vi "breakIn_toplvl_zapOption-v01.vi"(0 "Pressure box control in":T3={"Pressure box COM"="COM7", "pressure box type"=enum."ProportionAir", "High pos pressure (mBar)"=0.0, "Low pos pressure (mBar)"=0.0, "Vacuum pressure (mBar)"=0.0, "calibration"=enum."mightenRig"}, 1 "Multiclamp Handle In":u32=722860, 3 "which manipulator":T2(ring), 5 "break in duration (ms)":i32(knob)=100 min=50 max=2000 step=50 scale=0.0..2000.0, 7 "mclamp cluster":T1, 9 "give a zap?":bool, 11 "error in (no error)":errorcluster) -> (4 "Pressure box control out":T3, 15 "error out":errorcluster)   [LabVIEW 2015]
uses:
  controls/proportionAir_cmds.ctl
  controls/arduino_pressure_setting.ctl
  multiBot/patcherBot/AxMultiClampMsg.dll
  controls/pressure_box_type.ctl
  controls/pressure_box_control.ctl
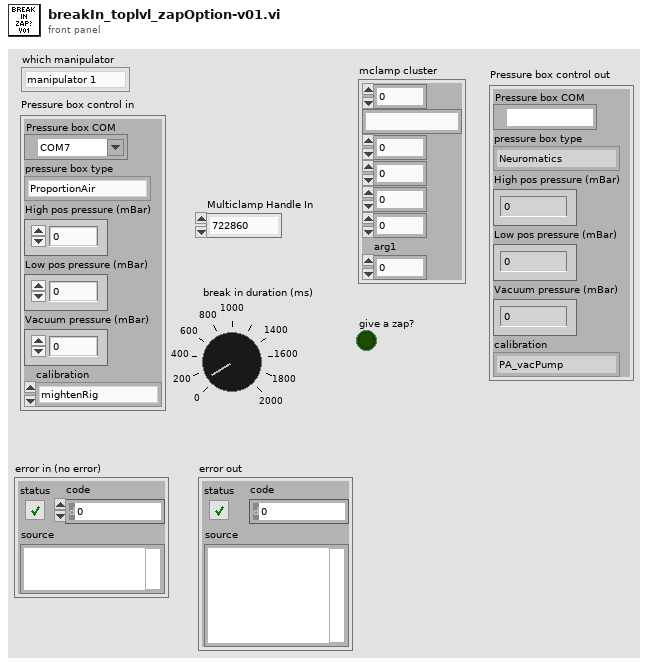
[diagram p1: front panel]
types:
  T1 = cluster{u32, string, i32, u32, u32, u32, "arg1":i32}
  T2 = enum16{"manipulator 1", "manipulator 2", "manipulator 3", "manipulator 4"}
  T3 = typedef "pressure_box_control.ctl" = cluster{"Pressure box COM":refnum<visa-resource-name>, "pressure box type":T4, "High pos pressure (mBar)":dbl, "Low pos pressure (mBar)":dbl, "Vacuum pressure (mBar)":dbl, "calibration":enum16{"PA_vacPump", "PA_venturi", "Neuromatics", "ilyaRig", "mightenRig"}}
  T4 = typedef "pressure_box_type.ctl" = enum16{"Neuromatics", "ProportionAir", "Demo box", "N-ProportionAir"}
  T5 = typedef "proportionAir_cmds.ctl" = enum16{"Set P", "Switch to Atm", "Switch to Regulator", "Pulse", "WC"}
  T6 = typedef "arduino_pressure_setting.ctl" = enum16{"High Positive Pressure", "Low Positive Pressure", "Atmospheric Pressure", "Low Vacuum", "High Vacuum", "Break In", "Puff"}
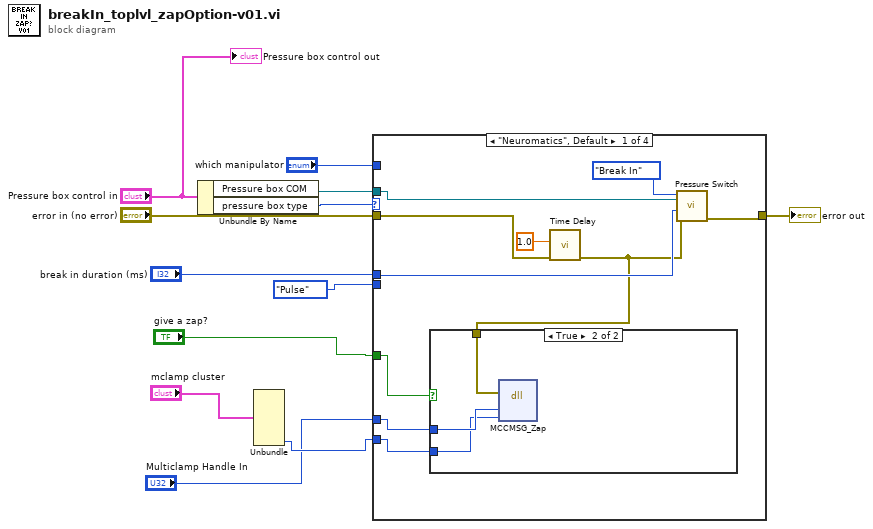
[diagram p0: block diagram]
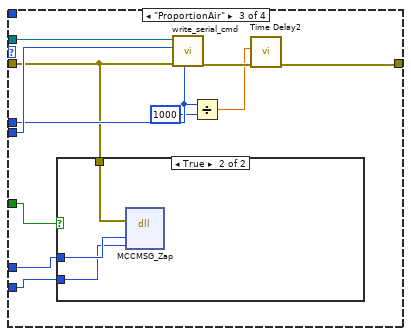
[diagram p4: hidden frame]
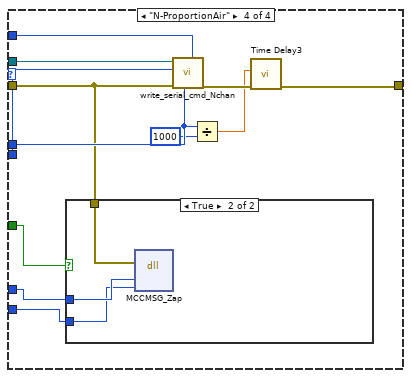
[diagram p6: hidden frame]
diagram:
  n1 = Unbundle By Name("Pressure box control in") -> ("Pressure box COM"=w10:refnum<visa-resource-name>, "pressure box type"=w11:T4)
  n2 = Unbundle("mclamp cluster") -> ("arg1"=w2:i32)  [unwired: 6 out]
  n3 = case shown="\"Neuromatics\", Default" w11 {
    tunnel: "error in (no error)" -> [w17 w26 w27 w41]
    tunnel: [w22 w26 w34 w49] -> w9
    tunnel: w10 -> [w18 _ w37 w52]
    tunnel: proportionAir_cmds."Pulse" ("pressure command") -> [_ _ w36 w51]
    tunnel: "break in duration (ms)" -> [w21 _ w33 w48]
    tunnel: "which manipulator" -> [_ _ _ w45]
    tunnel: "give a zap?" -> [w16 _ w28 w44]
    tunnel: w2 -> [w14 _ w29 w42]
    tunnel: "Multiclamp Handle In" -> [w15 _ w30 w43]
    frame "Neuromatics", Default {
      n4 = call "Time Delay"("error in (no error)"=w17, "Delay Time (s)"=1.0) -> ("error out"=w13:errorcluster)  [unwired: 9 in]
      n5 = case shown="True" w16 {
        tunnel: w15 -> [_ w25]
        tunnel: w14 -> [_ w24]
        tunnel: w13 -> [_ w23]
        frame False {
        }
        frame True {
          n6 = dll-call lib="C:/multiBot/patcherBot/AxMultiClampMsg.dll" fn="MCCMSG_Zap"(error in=w23, "handle"=w25, "error"=w24) -> ()  [unwired: 5 in, 2 out]
        }
      }
      n7 = call "Pressure Switch.vi"("error in"=w13, "Break In Time"=w21, "Pressure Box COM"=w18, "arduino pressure setting"=arduino_pressure_setting."Break In") -> ("error out"=w22:errorcluster)  [unwired: 6 in, 1 out]
    }
    frame "Demo box" {
    }
    frame "ProportionAir" {
      n8 = case shown="True" w28 {
        tunnel: w30 -> [_ w40]
        tunnel: w29 -> [_ w39]
        tunnel: w27 -> [_ w38]
        frame False {
        }
        frame True {
          n9 = dll-call lib="C:/multiBot/patcherBot/AxMultiClampMsg.dll" fn="MCCMSG_Zap"(error in=w38, "handle"=w40, "error"=w39) -> ()  [unwired: 5 in, 2 out]
        }
      }
      n10 = call "write_serial_cmd.vi"("pulse duration (ms)"=w33, "error in"=w27, "pressure command"=w36, "Pressure Box COM"=w37) -> ("error out"=w35:errorcluster)  [unwired: 6 in, 1 out]
      n11 = Divide(x=w33, y=1000) -> (x/y=w31:dbl)
      n12 = call "Time Delay2"("error in (no error)"=w35, "Delay Time (s)"=w31) -> ("error out"=w34:errorcluster)  [unwired: 9 in]
    }
    frame "N-ProportionAir" {
      n13 = case shown="True" w44 {
        tunnel: w43 -> [_ w55]
        tunnel: w42 -> [_ w54]
        tunnel: w41 -> [_ w53]
        frame False {
        }
        frame True {
          n14 = dll-call lib="C:/multiBot/patcherBot/AxMultiClampMsg.dll" fn="MCCMSG_Zap"(error in=w53, "handle"=w55, "error"=w54) -> ()  [unwired: 5 in, 2 out]
        }
      }
      n15 = call "write_serial_cmd_Nchan.vi"("which manipulator"=w45, "arg 2"=w48, "error in"=w41, "pressure command"=w51, "Pressure Box COM"=w52) -> ("error out"=w50:errorcluster)  [unwired: 5 in, 1 out]
      n16 = Divide(x=w48, y=1000) -> (x/y=w46:dbl)
      n17 = call "Time Delay3"("error in (no error)"=w50, "Delay Time (s)"=w46) -> ("error out"=w49:errorcluster)  [unwired: 9 in]
    }
  }
  "error out" <- w9
  "Pressure box control out" <- "Pressure box control in"
